vi "test_Create MetaData Channel_single channel type cast.vi"(8 "error in (no error)":errorcluster, 11 "TestCase in":refnum<class "Instrument Addon Scripting API Channels Unit Tests.lvclass">) -> (0 "error out":errorcluster, 3 "TestCase out":refnum<class "Instrument Addon Scripting API Channels Unit Tests.lvclass">)   [LabVIEW 2019, in "Instrument Addon Scripting API Channels Unit Tests.lvclass"]
uses:
  Instrument Addon Scripting API Channels Unit Tests.lvclass
  <vilib>/addons/_JKI Toolkits/VI Tester/TestCase.llb/TestCase.lvclass
  <vilib>/NI VeriStand/Custom Device Tools/Custom Device Utility Library/Custom Device Utility Library.lvlib
  Addon/Addon Shared/SubVIs/Constants.vi
  Addon/Addon Shared/Instrument Addon Shared.lvlib
  Addon/Addon Shared/Types/FG Control.ctl
  <vilib>/NI VeriStand/Custom Device API/Custom Device API.lvlib
  Addon/Addon Shared/Types/Type Cast Type.ctl
  Addon/Addon Shared/Types/Endian.ctl
  APIs/Scripting API/TypeDefs/Single Channel Type Cast Settings.ctl
  APIs/Scripting API/Instrument Addon Scripting API.lvlib
  <vilib>/NI VeriStand/Custom Device Tools/Custom Device Utility Library/NI VeriStand - Search for Item by Name.vi
  APIs/Scripting API/Channels/Create MetaData Channel - Single Channel - Type Cast.vi
  <vilib>/NI VeriStand/Custom Device Tools/Custom Device Utility Library/NI VeriStand - Search for Item by GUID.vi
  C:/Program Files (x86)/National Instruments/LabVIEW 2019/vi.lib/addons/_JKI Toolkits/VI Tester/TestCase.llb/TestCase.lvclass
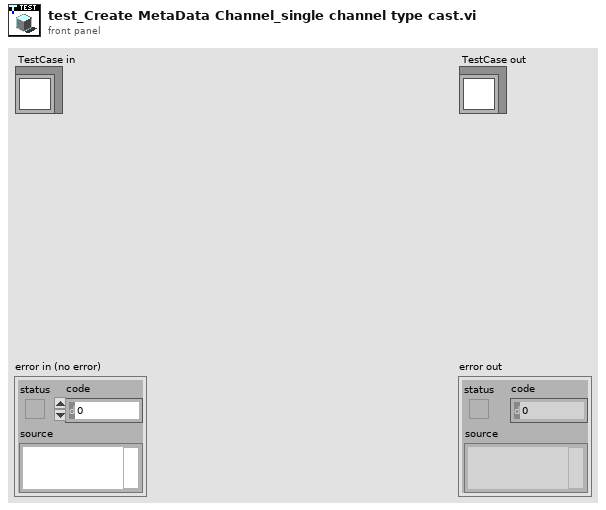
[diagram p1: front panel]
types:
  T1 = typedef "Instrument Addon Shared.lvlib/FG Control.ctl" = enum16{"Get", "Set"}
  T2 = typedef "Instrument Addon Scripting API.lvlib/Single Channel Type Cast Settings.ctl" = cluster{"Default Value":dbl, "Units":string, "Type":T3, "Endian":T4}
  T3 = typedef "Instrument Addon Shared.lvlib/Type Cast Type.ctl" = enum16{"DBL", "SGL", "U64", "U32", "U16", "U8", "I64", "I32", "I16", "I8"}
  T4 = typedef "Instrument Addon Shared.lvlib/Endian.ctl" = enum16{"Native", "Little", "Big"}
  T5 = typedef "Custom Device API.lvlib/Custom Device Item Ref.ctl" = u64
  T6 = typedef "Instrument Addon Shared.lvlib/MetaData Parameters.ctl" = cluster{"Data Type":T7, "Channel Type":T8, "List":string[], "Format String":string, "Type":T3, "Delimiter":string, "Endian":T4}
  T7 = typedef "Instrument Addon Shared.lvlib/Protocol Data Type.ctl" = enum16{"Single Channel", "Array"}
  T8 = typedef "Instrument Addon Shared.lvlib/Metadata Channel Type.ctl" = enum16{"Enumerated List", "Format", "Type Cast"}
  T9 = typedef "Custom Device API.lvlib/Custom Device Channel.ctl" = cluster{"Type":T10, "Units":string, "Default Value":dbl, "Faultable":bool, "Scalable":bool}
  T10 = typedef "Custom Device API.lvlib/Custom Device Channel Type.ctl" = enum16{"Input", "Output"}
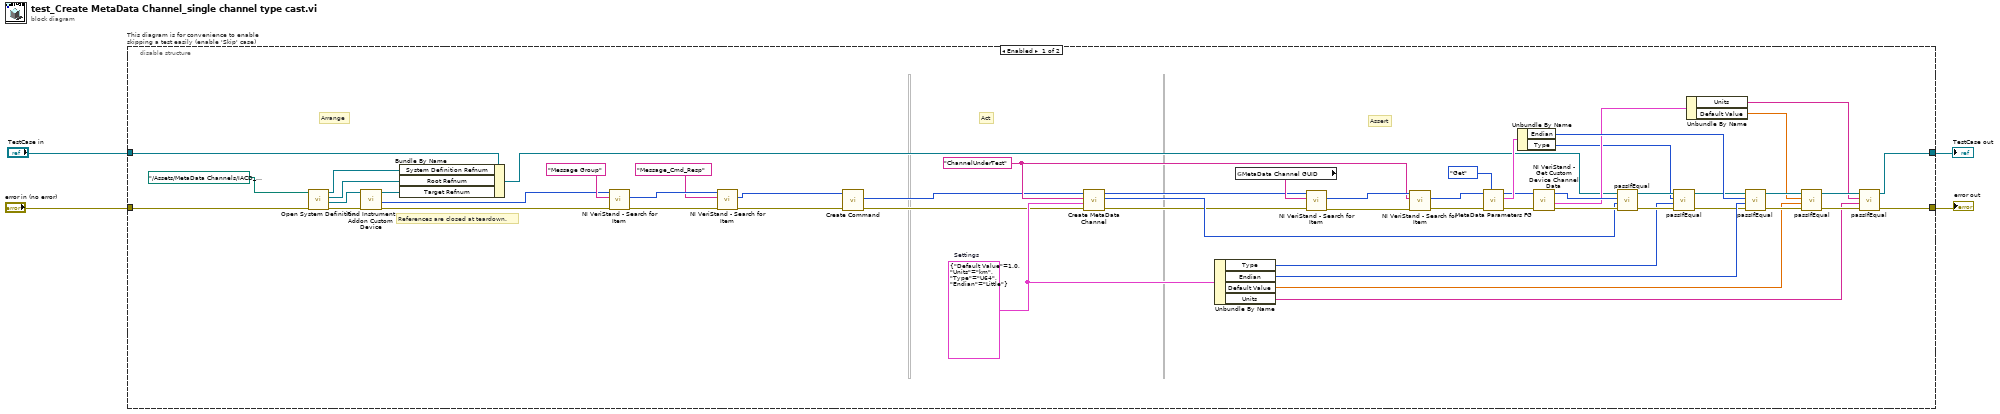
[diagram p0: block diagram]
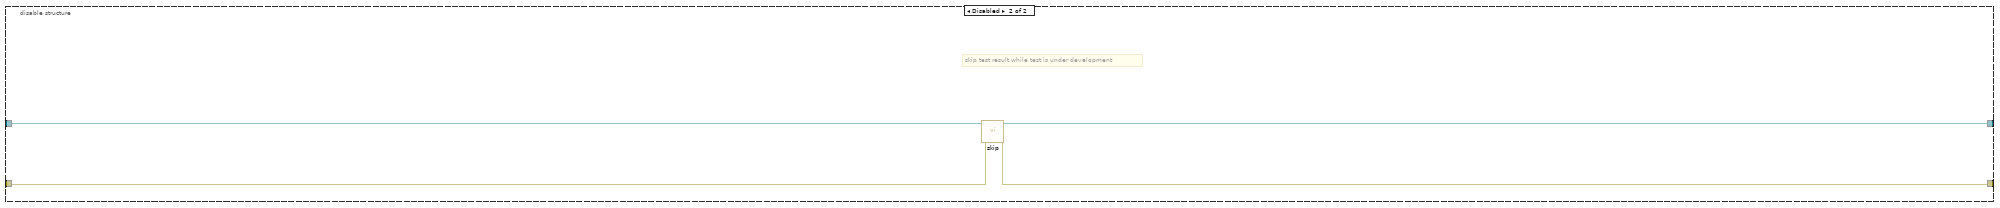
[diagram p2: hidden frame]
diagram:
  n1 = disable-structure "This diagram is for convenience to enable skipping a test easily (enable 'Skip' case)" shown="Enabled" {
    disable-tunnel: "TestCase in" -> [w27 w62]
    disable-tunnel: [w34 w60] -> w1
    disable-tunnel: [w33 w61] -> w3
    disable-tunnel: "error in (no error)" -> [w58 w59]
    frame Enabled {
      w13 = T2 {"Default Value"=1.0, "Units"="km", "Type"=enum."U64", "Endian"=enum."Little"}  # Settings
      w14 = "ChannelUnderTest" ("Name")
      # "References are closed at teardown."
      # "Assert"
      # "Act"
      # "Arrange"
      n2 = call "Open System Definition.vi"("error in (no error)"=w58, "System Definition File"=path "../Assets/MetaData Channels/IACD_channels.nivssdf") -> ("error out"=w56:errorcluster, "Target Refnum"=w57:refnum<k24>, "Root Refnum"=w30:refnum<k24>, "System Definition Refnum"=w29:refnum<k24>)  [unwired: 6 in]
      n3 = call "Find Instrument Addon Custom Device.vi"("error in"=w56, "target in"=w57) -> ("error out"=w16:errorcluster, "NodeID"=w15:u64, "target out"=w31:refnum<k24>)  [unwired: 7 in]
      n4 = Bundle By Name(cluster=w27, "System Definition Refnum"=w29, "Root Refnum"=w30, "Target Refnum"=w31) -> (w28:refnum<class "Instrument Addon Scripting API Channels Unit Tests.lvclass">)
      n5 = call-poly <vilib>:"NI VeriStand - Search for Item.vi"("error in"=w16, "Item Name"="Message Group", "Section Ref in"=w15) -> ("error out"=w17:errorcluster, "Item Ref"=w19:T5)  [unwired: 5 in, 2 out]
      n6 = call-poly <vilib>:"NI VeriStand - Search for Item.vi"("error in"=w17, "Item Name"="Message_Cmd_Resp", "Section Ref in"=w19) -> ("error out"=w8:errorcluster, "Item Ref"=w7:T5)  [unwired: 5 in, 2 out]
      n7 = call "Create Command.vi"("error in"=w8, "message refnum In"=w7) -> ("error out"=w5:errorcluster, "command refnum"=w6:T5)  [unwired: 7 in, 1 out]
      n8 = call-poly "Create MetaData Channel.vi"("error in (no error)"=w5, "settings"=w13, "channel name"=w14, "command refnum in"=w6) -> ("error out"=w10:errorcluster, "channel refnum"=w11:T5, "command refnum out"=w12:T5)  [unwired: 5 in]
      n9 = Unbundle By Name(w13) -> ("Type"=w22:T3, "Endian"=w43:T4, "Default Value"=w39:dbl, "Units"=w38:string)
      n10 = global read "Constants.vi" "MetaData Channel GUID"() -> (w55:string)
      n11 = call-poly <vilib>:"NI VeriStand - Search for Item.vi"("error in"=w10, "Item GUID"=w55, "Section Ref in"=w12) -> ("error out"=w53:errorcluster, "Item Ref"=w54:T5)  [unwired: 5 in, 2 out]
      n12 = call-poly <vilib>:"NI VeriStand - Search for Item.vi"("error in"=w53, "Item Name"=w14, "Section Ref in"=w54) -> ("error out"=w52:errorcluster, "Item Ref"=w51:T5)  [unwired: 5 in, 2 out]
      n13 = call "MetaData Parameters FG.vi"("Action"=FG_Control."Get", "error in (no error)"=w52, "Item Ref in"=w51) -> ("error out"=w41:errorcluster, "MetaData Parameters"=w49:T6, "Item Ref out"=w42:T5)  [unwired: 6 in]
      n14 = Unbundle By Name(w49) -> ("Endian"=w44:T4, "Type"=w21:T3)
      n15 = call <vilib>:"NI VeriStand - Get Custom Device Channel Data.vi"("error in (no error)"=w41, "Channel Ref in"=w42) -> ("error out"=w32:errorcluster, "Channel"=w37:T9, "Channel Ref out"=w40:T5)  [unwired: 4 in, 3 out]
      n16 = call-dynamic "passIfEqual.vi"("error in (no error)"=w32, "y"=w11, "x"=w40, "TestCase in"=w28) -> ("error out"=w26:errorcluster, "TestCase out"=w24:refnum<class "Instrument Addon Scripting API Channels Unit Tests.lvclass">)  [unwired: 6 in]
      n17 = call-dynamic "passIfEqual.vi"("error in (no error)"=w26, "y"=w22, "x"=w21, "TestCase in"=w24) -> ("error out"=w25:errorcluster, "TestCase out"=w23:refnum<class "Instrument Addon Scripting API Channels Unit Tests.lvclass">)  [unwired: 6 in]
      n18 = Unbundle By Name(w37) -> ("Units"=w35:string, "Default Value"=w36:dbl)
      n19 = call-dynamic "passIfEqual.vi"("error in (no error)"=w25, "y"=w43, "x"=w44, "TestCase in"=w23) -> ("error out"=w48:errorcluster, "TestCase out"=w47:refnum<class "Instrument Addon Scripting API Channels Unit Tests.lvclass">)  [unwired: 6 in]
      n20 = call-dynamic "passIfEqual.vi"("error in (no error)"=w48, "y"=w39, "x"=w36, "TestCase in"=w47) -> ("error out"=w46:errorcluster, "TestCase out"=w45:refnum<class "Instrument Addon Scripting API Channels Unit Tests.lvclass">)  [unwired: 6 in]
      n21 = call-dynamic "passIfEqual.vi"("error in (no error)"=w46, "y"=w38, "x"=w35, "TestCase in"=w45) -> ("error out"=w33:errorcluster, "TestCase out"=w34:refnum<class "Instrument Addon Scripting API Channels Unit Tests.lvclass">)  [unwired: 6 in]
    }
    frame Disabled {
      # "skip test result while test is under development"
      n22 = call <vilib>:"skip.vi"("error in (no error)"=w59, "TestCase in"=w62) -> ("error out"=w61:errorcluster, "TestCase out"=w60:refnum<class "Instrument Addon Scripting API Channels Unit Tests.lvclass">)  [unwired: 8 in]
    }
  }
  "error out" <- w3
  "TestCase out" <- w1
